vi "gc-zyklus mfc mpos konfig sub.vi"() -> ()   [LabVIEW 2010]
uses:
  <vilib>/Instr/_visa.llb/VISA Configure Serial Port (Instr).vi
panel:
  in  "Konfigurationsdatei auswählen":path
  out "Konfiguration":string
  out "Zeitpunkt":string
  out "Temperatur (°C)":u16
  out "Meßwert PC2 (mbara)":u16
  out "Meßwert PC1 (mbara)":u16
  out "Meßwert FC (mln/min)":u16
  in  "Setpoint PC1 (bara)":dbl min=0.15 max=3.0 step=0.05
  in  "Setpoint PC2 (bara)":dbl min=0.15 max=3.0 step=0.05
  in  "Messwerte speichern":path
  out "Zyklus Nr.":i32
  out "Positionen (1-6)":i32[](array[numeric])=[1, 3, 5, 2]
  out "Anzahl der Zustände (Mpos.-Ventil)":i32
  out "aktuelle Position":i32
  out "Setpoints FC (ln/min)":dbl[](array[numeric])=[1.0, 3.0, 5.0, 2.0]
  out "Längen der Zustände (s)":i32[](array[numeric])=[1, 3, 5, 2]
  out "Anzahl der Zustände (MFC)":i32
  out "Länge des aktuellen Zustandes (s)":i32
  out "aktueller Setpoint FC (ln/min)":dbl
  out "Sequenz Nr.":i32
  out "Aktuelle Zeit":timestamp
  in  "(Sequenz wird zu Ende geführt)":bool
  # "Gerät im Chromatographie-Zyklus, z.B. MFC"
  # "Multipositionsventil"
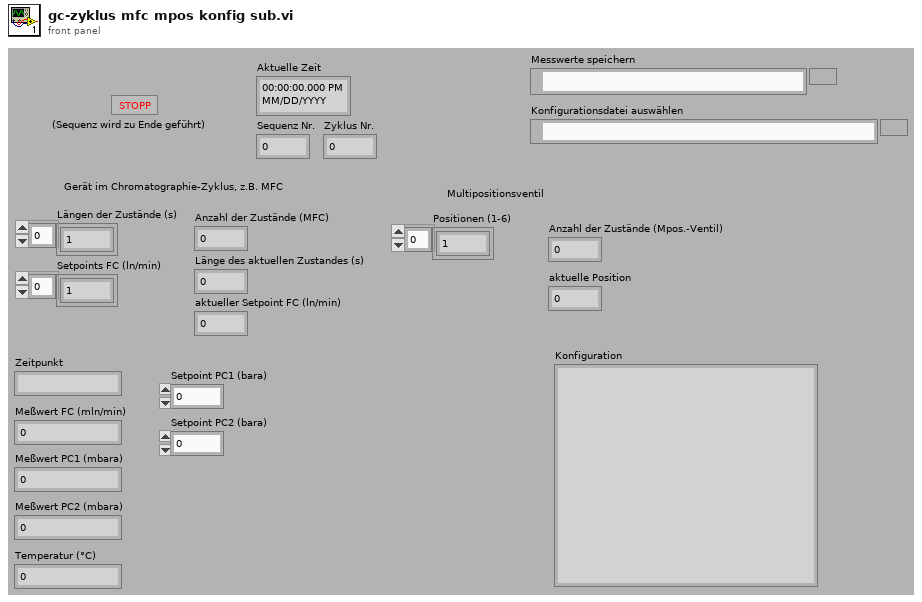
[diagram p1: front panel]
types:
  T1 = enum16{"open", "replace", "create", "open or create", "replace or create", "replace or create with confirmation"}
  T2 = cluster{"Mode":enum16{"RTU", "ASCII"}, "Slave Address":u8}
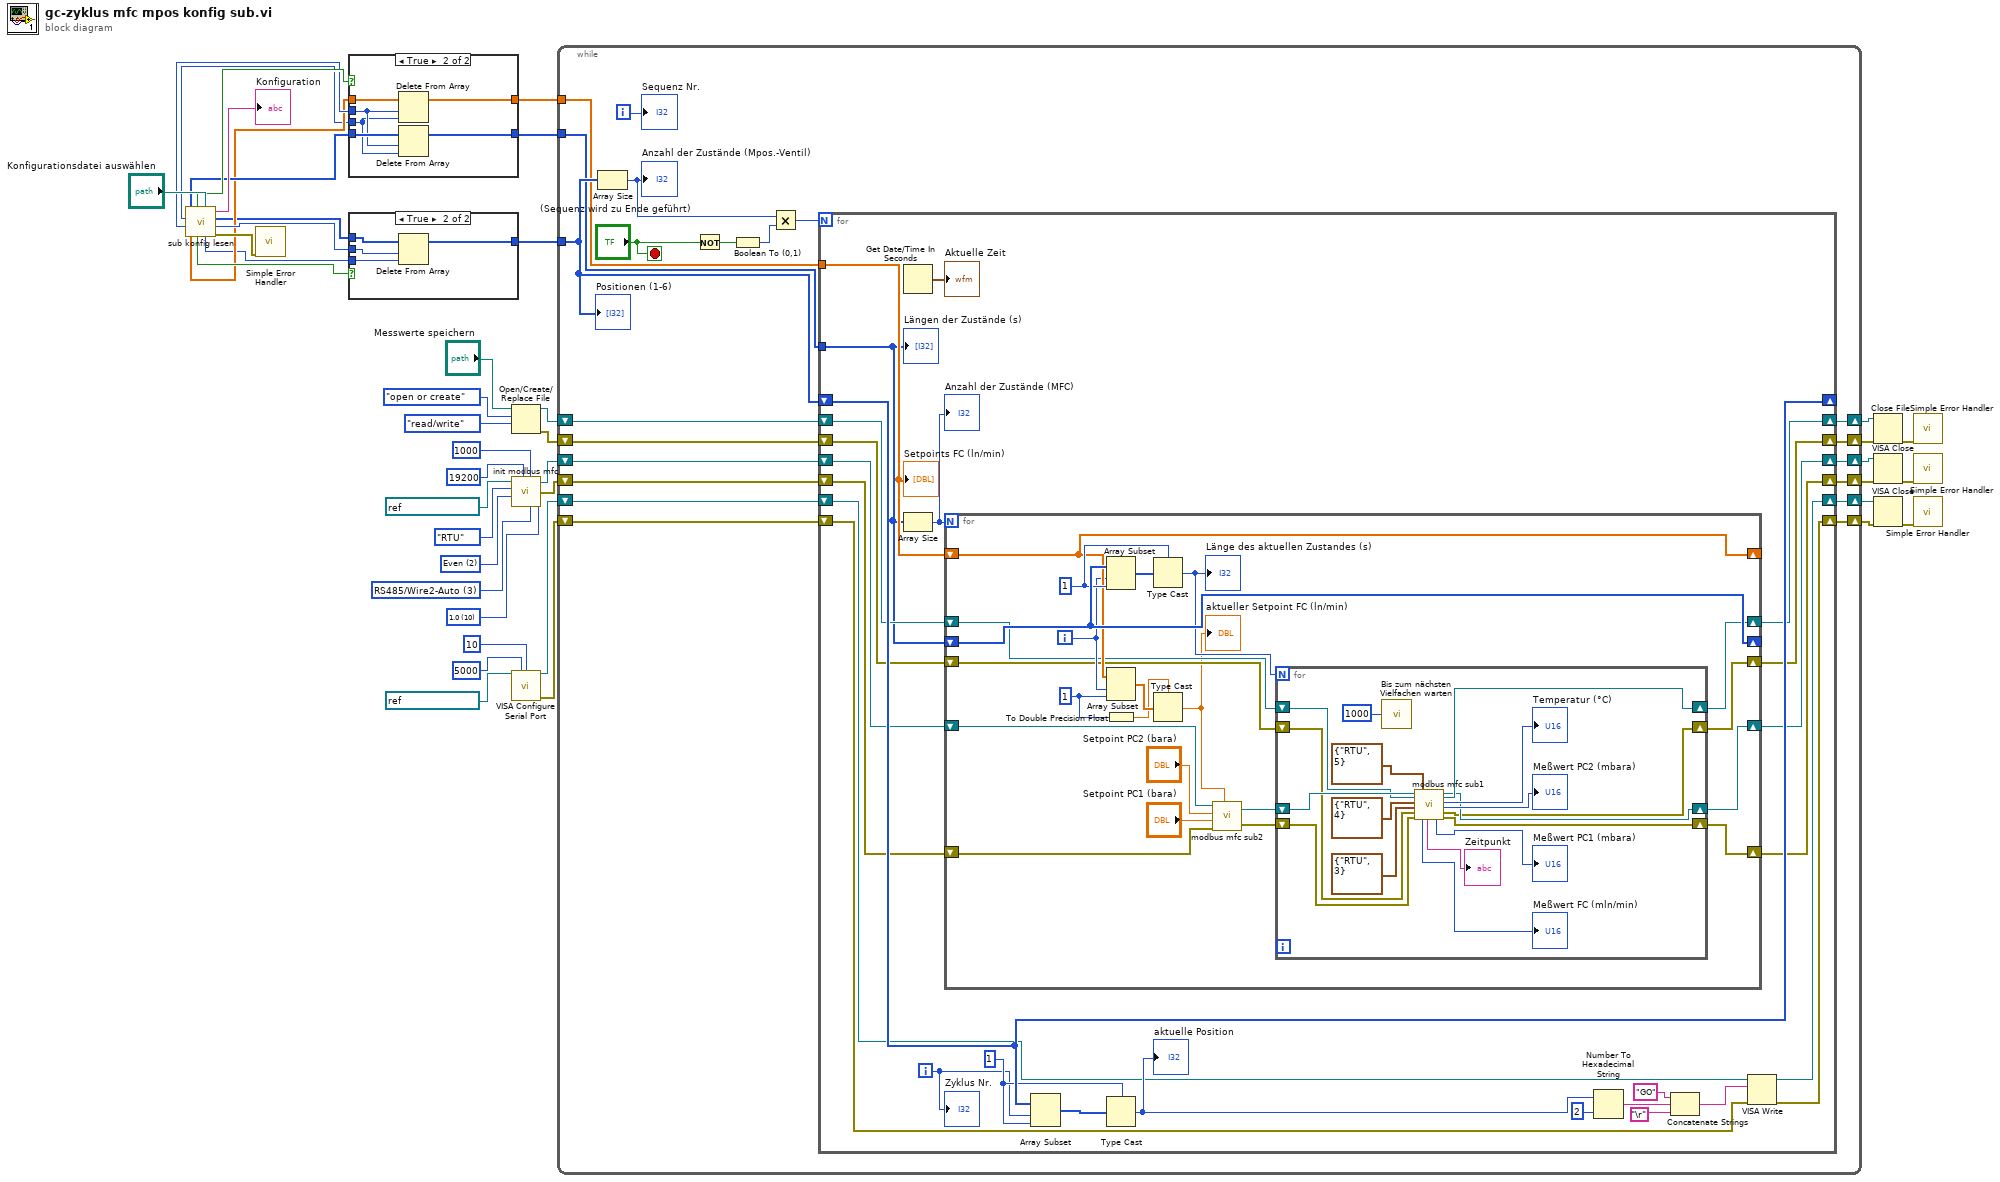
[diagram p0: block diagram]
diagram:
  w40 = u16 10 items=["1.0"=10, "1.5"=15, "2.0"=20] ("Serial Settings:Stop Bits")
  w38 = u16 2 items=["None", "Odd", "Even", "Mark", "Space"] ("Parity")
  w39 = i16 3 items=["Unknown"=-1, "RS485/Wire4"=0, "RS485/Wire2-EchoDTR"=1, "RS485/Wire2-CtrlDTR"=2, "RS485/Wire2-Auto"=3, "RS232/DTE"=128, "RS232/DCE"=129, "RS232/AUTO"=130] ("Serial Settings:Wire Mode")
  n1 = call "sub konfig lesen.vi"("Konfigurationsdatei auswählen"="Konfigurationsdatei auswählen") -> ("error out"=w15:errorcluster, "Numerisch 4"=w11:i32, "Array"=w6:i32[], "String"=→"Konfiguration":string, "Numerisch 2"=w5:i32, "Boolesch 2"=w12:bool, "Boolesch"=w10:bool, "Array 2"=w7:dbl[], "Numerisch 3"=w9:i32, "Numerisch"=w4:i32, "Array 3"=w8:i32[])
  n2 = call <vilib>:"Simple Error Handler.vi"("error in (no error)"=w15) -> ()  [unwired: 4 in, 5 out]
  n3 = case shown="True" w10 {
    tunnel: w8 -> [w45 w51]
    tunnel: w4 -> [_ w46]
    tunnel: [w45 w50] -> w1
    tunnel: w9 -> [_ w47]
    tunnel: w7 -> [w44 w49]
    tunnel: [w44 w48] -> w2
    frame False {
    }
    frame True {
      n4 = Delete From Array(array=w49, length=w47, index=w46) -> (array with subset deleted=w48:dbl[])  [unwired: 1 out]
      n5 = Delete From Array(array=w51, length=w47, index=w46) -> (array with subset deleted=w50:i32[])  [unwired: 1 out]
    }
  }
  n6 = case shown="True" w12 {
    tunnel: w6 -> [w52 w56]
    tunnel: w5 -> [_ w54]
    tunnel: [w52 w55] -> w3
    tunnel: w11 -> [_ w53]
    frame False {
    }
    frame True {
      n7 = Delete From Array(array=w56, length=w53, index=w54) -> (array with subset deleted=w55:i32[])  [unwired: 1 out]
    }
  }
  n8 = Open/Create/Replace File(file path (use dialog)="Messwerte speichern", operation (0:open)=T1."open or create" ("Operation (0:Öffnen)"), access (0:read/write)=enum16{"read/write", "read-only", "write-only"}."read/write" ("Zugriff (0:Lesen/Schreiben)")) -> (refnum out=w33:refnum<file>, error out=w32:errorcluster)  [unwired: 3 in, 1 out]
  n9 = call "init modbus mfc.vi"("Timeout"=u32 1000, "Serial Settings:Stop Bits"=w40, "Serial Settings:Wire Mode"=w39, "Baud Rate"=u32 19200, "VISA resource name"=refnum<visa-resource-name> "ASRL2::INSTR", "Mode"=enum16{"RTU", "ASCII"}."RTU", "Parity"=w38) -> ("VISA resource name out"=w31:refnum<visa-resource-name>, "error out"=w30:errorcluster)  [unwired: 2 in]
  n10 = call-poly "VISA Configure Serial Port"("VISA resource name"=refnum<visa-resource-name> "ASRL1::INSTR", "timeout (10sec)"=u32 5000, "termination char\n(0xA = '\\n' = LF)"=u8 10 ("termination char\n(0xA = '\\n' = LF)")) -> ("VISA resource name out"=w20:refnum<visa-resource-name>, "error out"=w19:errorcluster)  [unwired: 11 in]
  n11 = while {
    shift-right: [w67] -> w24
    shift-left: w33 -> [w71]
    shift-right: [w66] -> w23
    shift-left: w32 -> [w70]
    shift-right: [w65] -> w22
    shift-left: w31 -> [w69]
    shift-right: [w64] -> w21
    shift-left: w30 -> [w68]
    shift-right: [w61] -> w17
    shift-left: w20 -> [w63]
    shift-right: [w60] -> w16
    shift-left: w19 -> [w62]
    tunnel: w3 -> [w59]
    tunnel: w2 -> [w58]
    tunnel: w1 -> [w57]
    i -> [w77]
    stop <- "(Sequenz wird zu Ende geführt)" stop-if-true
    n12 = Array Size(array=w59) -> (size(s)=w76:i32)
    "Anzahl der Zustände (Mpos.-Ventil)" <- w76
    n13 = Not(x="(Sequenz wird zu Ende geführt)") -> (.not. x?=w74:bool)
    n14 = Boolean To (0,1)(Boolean=w74) -> (0, 1=w72:i16)
    n15 = Multiply(x=w76, y=w72) -> (x*y=w73:i32)
    n16 = for {
      N: w73 -> [_]
      shift-right: [w103] -> _
      shift-left: w59 -> [w103]
      shift-right: [w87] -> w67
      shift-left: w71 -> [w95]
      shift-right: [w86] -> w66
      shift-left: w70 -> [w96]
      shift-right: [w85] -> w65
      shift-left: w69 -> [w98]
      shift-right: [w84] -> w64
      shift-left: w68 -> [w97]
      shift-right: [w81] -> w61
      shift-left: w63 -> [w83]
      shift-right: [w80] -> w60
      shift-left: w62 -> [w82]
      tunnel: w58 -> [w79]
      tunnel: w57 -> [w78]
      i -> [w100]
      w102 = 1 ("Länge")
      n17 = Get Date/Time In Seconds() -> (seconds since 1Jan1904=→"Aktuelle Zeit":timestamp)
      n18 = Array Size(array=w78) -> (size(s)=w94:i32)
      "Anzahl der Zustände (MFC)" <- w94
      n19 = for {
        N: w94 -> [_]
        shift-right: [w125] -> _
        shift-left: w78 -> [w125]
        shift-right: [w121] -> _
        shift-left: w79 -> [w121]
        shift-right: [w114] -> w87
        shift-left: w95 -> [w115]
        shift-right: [w112] -> w86
        shift-left: w96 -> [w116]
        shift-right: [w113] -> w85
        shift-left: w98 -> [w107]
        shift-right: [w111] -> w84
        shift-left: w97 -> [w106]
        i -> [w120]
        w118 = 1 ("Länge")
        w124 = 1 ("Länge")
        n20 = Array Subset(array=w125, index=w120, length=w124) -> (w123:i32[])
        n21 = Array Subset(array=w121, index=w120, length=w118) -> (w122:dbl[])
        n22 = To Double Precision Float(number=w118) -> (double precision float=w117:dbl)
        n23 = Type Cast(type=w124, x=w123) -> (*(type *) &x=w119:i32)
        "Länge des aktuellen Zustandes (s)" <- w119
        n24 = Type Cast(type=w117, x=w122) -> (*(type *) &x=w108:dbl)
        "aktueller Setpoint FC (ln/min)" <- w108
        n25 = call "modbus mfc sub2.vi"("VISA resource name out 2"=w107, "Setpoint PC2 (bara)"="Setpoint PC2 (bara)", "Setpoint PC1 (bara)"="Setpoint PC1 (bara)", "error out 2"=w106, "Setpoint FC (ln/min)"=w108) -> ("VISA resource name out"=w105:refnum<visa-resource-name>, "error out"=w104:errorcluster)
        n26 = for {
          N: w119 -> [_]
          shift-right: [w128] -> w113
          shift-left: w105 -> [w132]
          shift-right: [w129] -> w114
          shift-left: w115 -> [w130]
          shift-right: [w127] -> w112
          shift-left: w116 -> [w131]
          shift-right: [w126] -> w111
          shift-left: w104 -> [w133]
          n27 = call "Bis zum nächsten Vielfachen warten"("Count(mSec)"=u32 1000) -> ()  [unwired: 1 out]
          n28 = call "modbus mfc sub1.vi"("VISA resource name out"=w132, "refnum out 2"=w130, "Serial Parameters 2"=T2 {"Mode"=enum."RTU", "Slave Address"=4}, "Serial Parameters"=T2 {"Mode"=enum."RTU", "Slave Address"=3}, "error out 2"=w131, "error out 3"=w133, "Serial Parameters 3"=T2 {"Mode"=enum."RTU", "Slave Address"=5}) -> ("Numerisch 3"=→"Meßwert FC (mln/min)":u16, "date/time string"=→"Zeitpunkt":string, "Numerisch 2"=→"Meßwert PC1 (mbara)":u16, "VISA resource name out 2"=w128:refnum<visa-resource-name>, "refnum out"=w129:refnum<file>, "Numerisch 4"=→"Temperatur (°C)":u16, "Numerisch"=→"Meßwert PC2 (mbara)":u16, "error out"=w127:errorcluster, "error out 4"=w126:errorcluster)  [unwired: 3 in, 1 out]
        }
      }
      n29 = Array Subset(array=w103, index=w100, length=w102) -> (w101:i32[])
      n30 = Type Cast(type=w102, x=w101) -> (*(type *) &x=w88:i32)
      "aktuelle Position" <- w88
      n31 = Number To Hexadecimal String(1:i16 2 ("Breite (-)"), 2:w88) -> (0:w92:string)
      n32 = Concatenate Strings("GO" ("String"), w92, "\r") -> (w93:string)
      n33 = VISA Write(VISA resource name=w83, write buffer=w93, error in (no error)=w82) -> (VISA resource name out=w81:refnum<visa-resource-name>, error out=w80:errorcluster)  [unwired: 1 out]
      "Längen der Zustände (s)" <- w78
      "Setpoints FC (ln/min)" <- w79
      "Zyklus Nr." <- w100
    }
    "Positionen (1-6)" <- w59
    "Sequenz Nr." <- w77
  }
  n34 = Close File(refnum=w24, error in=w23) -> (error out=w28:errorcluster)  [unwired: 1 out]
  n35 = VISA Close(VISA resource name=w22, error in (no error)=w21) -> (error out=w29:errorcluster)
  n36 = VISA Close(VISA resource name=w17, error in (no error)=w16) -> (error out=w18:errorcluster)
  n37 = call <vilib>:"Simple Error Handler.vi"("error in (no error)"=w28) -> ()  [unwired: 4 in, 5 out]
  n38 = call <vilib>:"Simple Error Handler.vi"("error in (no error)"=w29) -> ()  [unwired: 4 in, 5 out]
  n39 = call <vilib>:"Simple Error Handler.vi"("error in (no error)"=w18) -> ()  [unwired: 4 in, 5 out]
